vi "Serialize Data.vi"(8 "error in (no error)":errorcluster, 11 "Process Data":T1) -> (0 "error out":errorcluster, 3 "Flat Data out":string)   [LabVIEW 2020, in "Optitrack.lvlib"]
doc: "Version 0.1"
uses:
  <vilib>/ADAS Record/CustomDataTypes/Optitrack/Optitrack.lvlib
  69b4f655-d322-486f-8d65-ee31f7d8c6ef.vi
  <vilib>/ADAS Record/IODataPEF/CfgMgr/FlatFormat.ctl
  <vilib>/ADAS Record/CustomDataTypes/Optitrack/Process Data.ctl
  Projects/NI AzDO/Mercedes-MPIC-201077/Record_MPIC3/mercedes-record-mpic3-201077/software-record-plugins/labview-2020/src/shared/TypeDef-Optitrack-RigidBody.ctl
  Projects/NI AzDO/Mercedes-MPIC-201077/Record_MPIC3/mercedes-record-mpic3-201077/software-record-plugins/labview-2020/src/shared/TypeDef-Optitrack-MarkerPoint.ctl
  Projects/NI AzDO/Mercedes-MPIC-201077/Record_MPIC3/mercedes-record-mpic3-201077/software-record-plugins/labview-2020/src/shared/TypeDef-Optitrack-MarkerSet.ctl
  Projects/NI AzDO/Mercedes-MPIC-201077/Record_MPIC3/mercedes-record-mpic3-201077/software-record-plugins/labview-2020/src/shared/TypeDef-Optitrack-LabeledMarker.ctl
  Projects/NI AzDO/Mercedes-MPIC-201077/Record_MPIC3/mercedes-record-mpic3-201077/software-record-plugins/labview-2020/src/shared/TypeDef-Optitrack-TrackedData.ctl
  Projects/NI AzDO/Mercedes-MPIC-201077/Record_MPIC3/mercedes-record-mpic3-201077/software-record-plugins/labview-2020/src/shared/TypeDef-Optitrack-FrameData.ctl
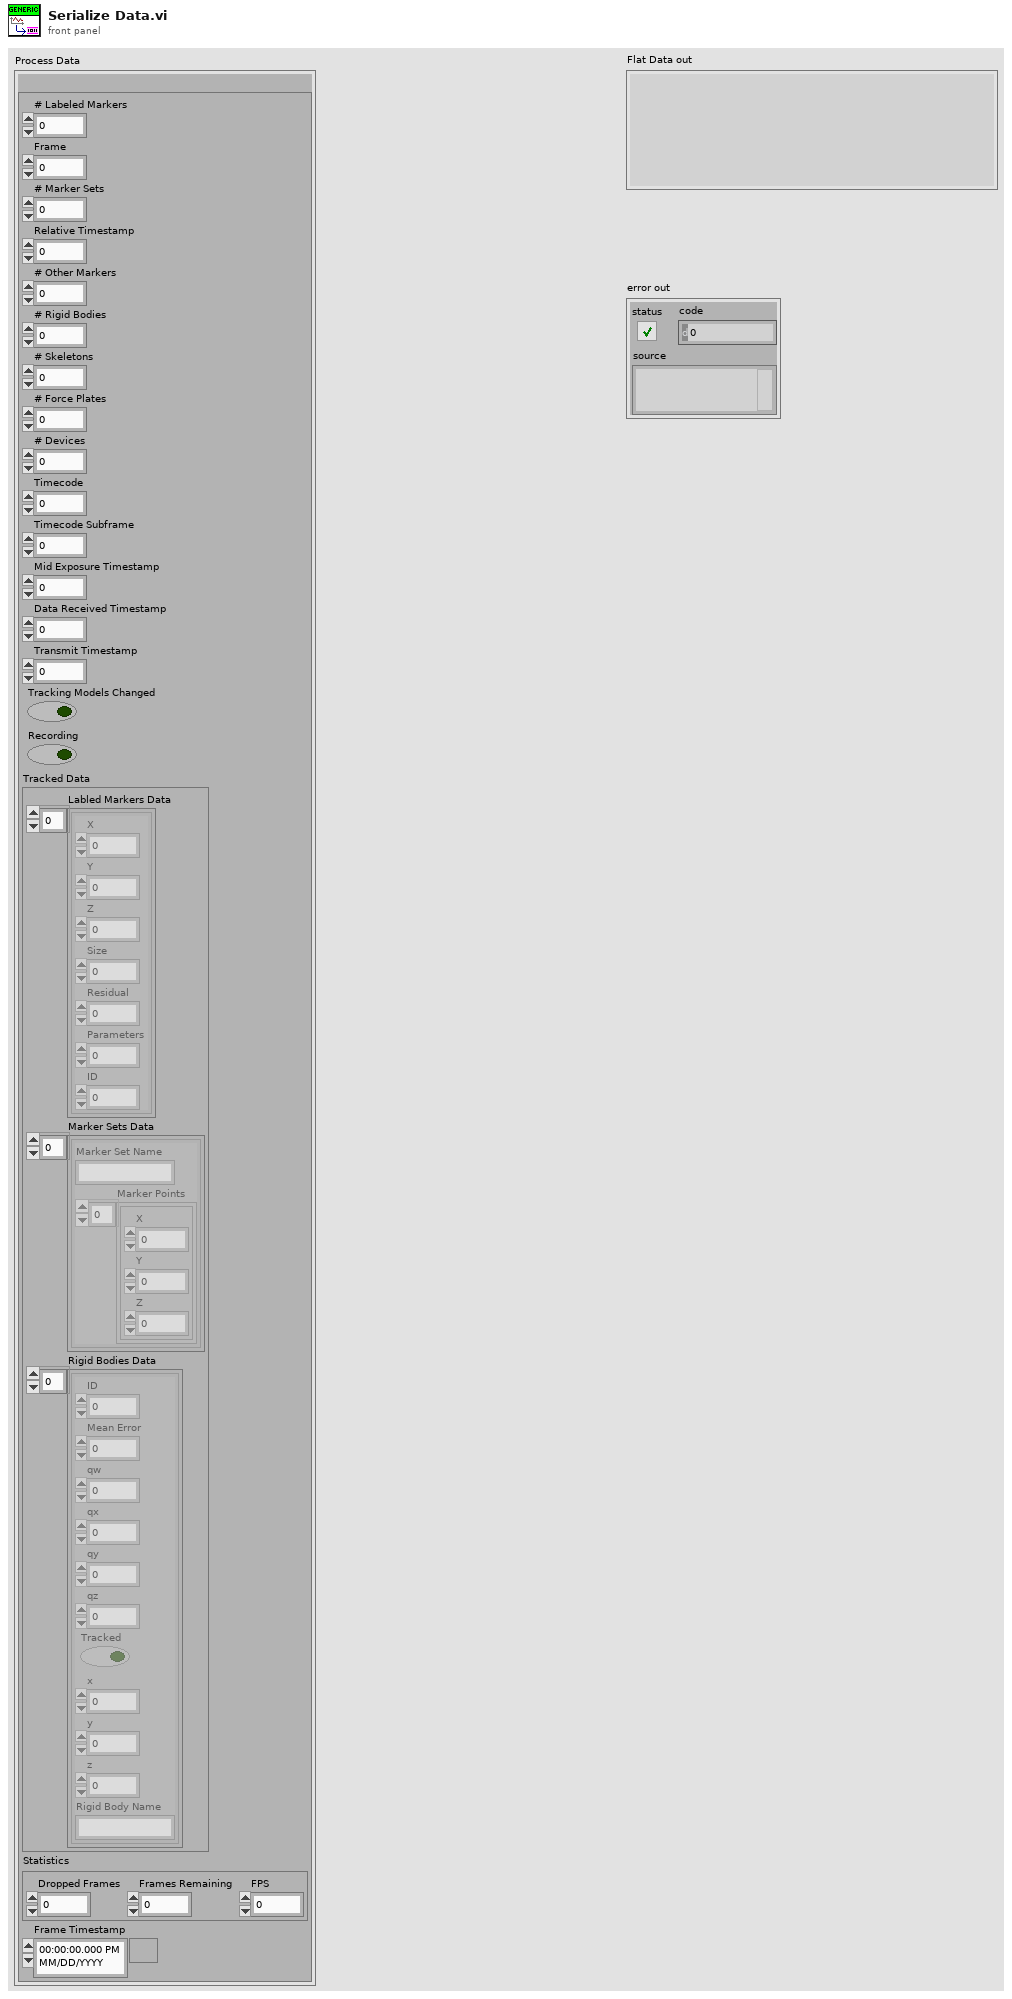
[diagram p1: front panel]
types:
  T1 = typedef "Optitrack.lvlib/Process Data.ctl" = cluster{"OptitrackFrame":T2}
  T2 = typedef "TypeDef-Optitrack-FrameData.ctl" = cluster{"# Labeled Markers":i32, "Frame":i32, "# Marker Sets":i32, "Relative Timestamp":dbl, "# Other Markers":i32, "# Rigid Bodies":i32, "# Skeletons":i32, "# Force Plates":i32, "# Devices":i32, "Timecode":u32, "Timecode Subframe":u32, "Mid Exposure Timestamp":u64, "Data Received Timestamp":u64, "Transmit Timestamp":u64, "Tracking Models Changed":bool, "Recording":bool, "Tracked Data":T3, "Statistics":cluster{"Dropped Frames":i32, "Frames Remaining":i32, "FPS":dbl}, "Frame Timestamp":timestamp}
  T3 = typedef "TypeDef-Optitrack-TrackedData.ctl" = cluster{"Labled Markers Data":T4[], "Marker Sets Data":T5[], "Rigid Bodies Data":T7[]}
  T4 = typedef "TypeDef-Optitrack-LabeledMarker.ctl" = cluster{"X":sgl, "Y":sgl, "Z":sgl, "Size":sgl, "Residual":sgl, "Parameters":i16, "ID":i32}
  T5 = typedef "TypeDef-Optitrack-MarkerSet.ctl" = cluster{"Marker Set Name":string, "Marker Points":T6[]}
  T6 = typedef "TypeDef-Optitrack-MarkerPoint.ctl" = cluster{"X":sgl, "Y":sgl, "Z":sgl}
  T7 = typedef "TypeDef-Optitrack-RigidBody.ctl" = cluster{"ID":i32, "Mean Error":sgl, "qw":sgl, "qx":sgl, "qy":sgl, "qz":sgl, "Tracked":bool, "x":sgl, "y":sgl, "z":sgl, "Rigid Body Name":string}
  T8 = typedef "FlatFormat.ctl" = enum32{"Auto", "PEF", "GFB (Apache)", "GFB", "JSON", "Readable JSON", "LV String", "Reserved", "LV Native"}
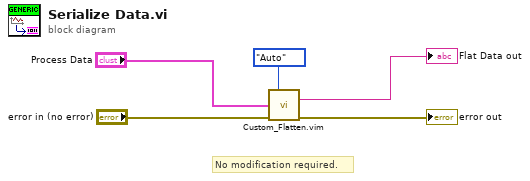
[diagram p0: block diagram]
diagram:
  # "No modification required."
  n1 = call "Custom_Flatten.vim"("Flat Format"=FlatFormat."Auto", "Data"="Process Data", "error in (no error)"="error in (no error)") -> ("Flat Data"=→"Flat Data out":string, "Error (out)"=→"error out":errorcluster)  [unwired: 10 in, 1 out]
